vi "Chi-Squared (Non-Central) Random.vi"(6 "seed":i32=-1, 7 "reset":bool, 9 "d":dbl, 10 "k":i32=1, 11 "samples":i32=128) -> (0 "error":i32, 3 "chi-squared(nc) random data":dbl[](array[numeric]))   [LabVIEW 2014, in "NI_Gmath.lvlib"]
doc: "Generates random values from a variate X, where X describes the selected distribution type. You must manually select the polymorphic instance to use."
uses:
  NI_Gmath.lvlib
panel:
  # "Chi-Squared (Non-Central) Random"
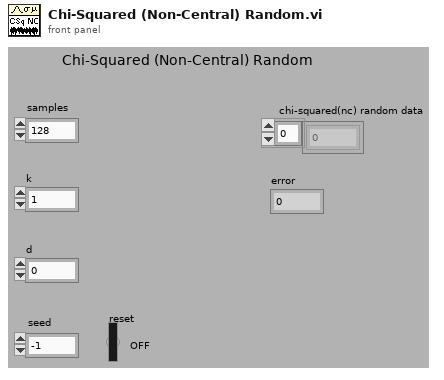
[diagram p1: front panel]
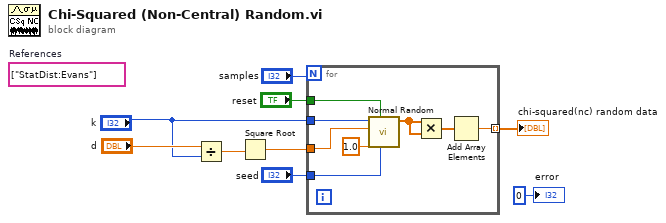
[diagram p0: block diagram]
diagram:
  (unwired) string[] ["StatDist:Evans"]  # References
  n1 = Divide(x="d", y="k") -> (x/y=w2:dbl)
  n2 = Square Root(x=w2) -> (sqrt(x)=w1:dbl)
  n3 = for {
    N: "samples" -> [_]
    tunnel: "k" -> [w14]
    tunnel: "seed" -> [w17]
    tunnel: [w16] -> w7 mode=indexing
    tunnel: "reset" -> [w11]
    tunnel: w1 -> [w10]
    n4 = call "Normal Random.vi"("seed"=w17, "reset"=w11, "std"=1.0, "mean"=w10, "samples"=w14) -> ("normal random data"=w13:dbl[])  [unwired: 5 in, 1 out]
    n5 = Multiply(x=w13, y=w13) -> (x*y=w12:dbl[])
    n6 = Add Array Elements(numeric array=w12) -> (sum=w16:dbl)
  }
  "chi-squared(nc) random data" <- w7
  "error" <- 0 ("error")
